vi "objectivesRegistrationMap.vi"   [LabVIEW 2017]
uses:
  39e2dec2-add2-4b11-9da2-3cbb0bf56f4d.vi
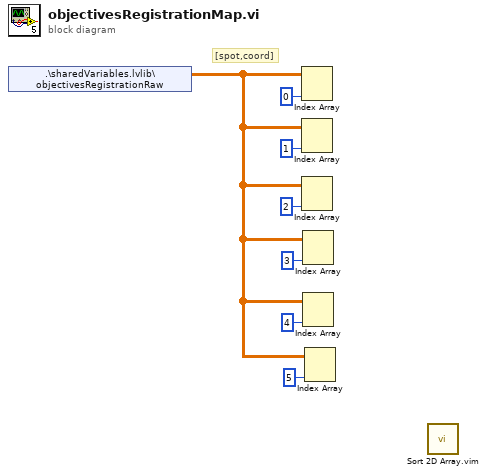
[diagram p0: block diagram]
diagram:
  # "[spot,coord]"
  n1 = shared-variable ".\\sharedVariables.lvlib\\objectivesRegistrationRaw"() -> (w1:dbl[][])  [unwired: 1 in, 1 out]
  n2 = Index Array(array=w1, index (col)=0 ("disabled index (col)")) -> ()  [unwired: 1 in, 1 out]
  n3 = Index Array(array=w1, index (col)=1 ("disabled index (col)")) -> ()  [unwired: 1 in, 1 out]
  n4 = Index Array(array=w1, index (col)=2 ("disabled index (col)")) -> ()  [unwired: 1 in, 1 out]
  n5 = Index Array(array=w1, index (col)=3 ("disabled index (col)")) -> ()  [unwired: 1 in, 1 out]
  n6 = Index Array(array=w1, index (col)=4 ("disabled index (col)")) -> ()  [unwired: 1 in, 1 out]
  n7 = Index Array(array=w1, index (col)=5 ("disabled index (col)")) -> ()  [unwired: 1 in, 1 out]
  n8 = call "Sort 2D Array.vim"() -> ()  [unwired: 10 in, 2 out]
